vi "ZufälligerDruck.vi"() -> (3 "Current Pressure":dbl)   [LabVIEW 2018]
uses:
  RT/[GlobVar]SensorState.vi
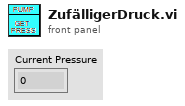
[diagram p1: front panel]
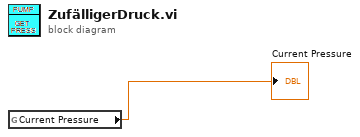
[diagram p0: block diagram]
diagram:
  n1 = global read "[GlobVar]SensorState.vi" "Current Pressure"() -> (→"Current Pressure":dbl)
